vi "dfd_Estimate Num of Bins from Order.vi"(10 "order":i32, 11 "# freq bins in":i32) -> (3 "# freq bins out":i32)   [LabVIEW 2017, in "NI_DigFilterLicensed.lvlib"]
uses:
  <vilib>/addons/Digital Filter Design/NI_DigFilterLicensed.lvlib
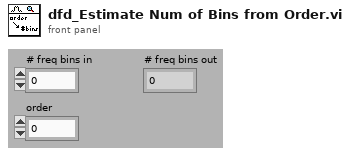
[diagram p1: front panel]
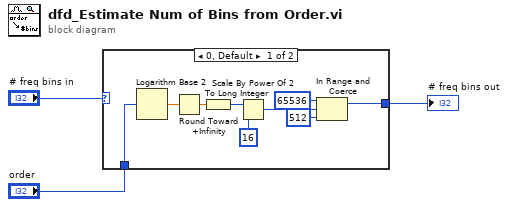
[diagram p0: block diagram]
diagram:
  n1 = case shown="0, Default" "# freq bins in" {
    selector: "# freq bins in" -> [_ w13]
    tunnel: "order" -> [w12 _]
    tunnel: [w8 w13] -> w2
    frame 0, Default {
      n2 = Logarithm Base 2(1:w12) -> (0:w11:dbl)
      n3 = Round Toward +Infinity(x=w11) -> (ceil(x): smallest int >= x=w10:dbl)
      n4 = To Long Integer(number=w10) -> (32bit integer=w7:i32)
      n5 = Scale By Power Of 2(n=w7, x=16) -> (x*2^n=w6:i32)
      n6 = In Range and Coerce(upper limit=65536, x=w6, lower limit=512 ("x")) -> (coerced(x)=w8:i32)  [unwired: 1 out]
    }
    frame 1.. {
    }
  }
  "# freq bins out" <- w2
